vi "Idle.vi"(8 "error in":errorcluster, 11 "VISA Interface in":refnum<class "VISA Interface.lvclass">) -> (0 "error out":errorcluster, 3 "VISA Interface out":refnum<class "VISA Interface.lvclass">)   [LabVIEW 2020, in "Plugin Instrument Driver.lvlib" / "VISA Interface.lvclass"]
doc: "Clears the buffer until all other configured Plugins are completed executing their initialize states"
uses:
  VISA Interface.lvclass
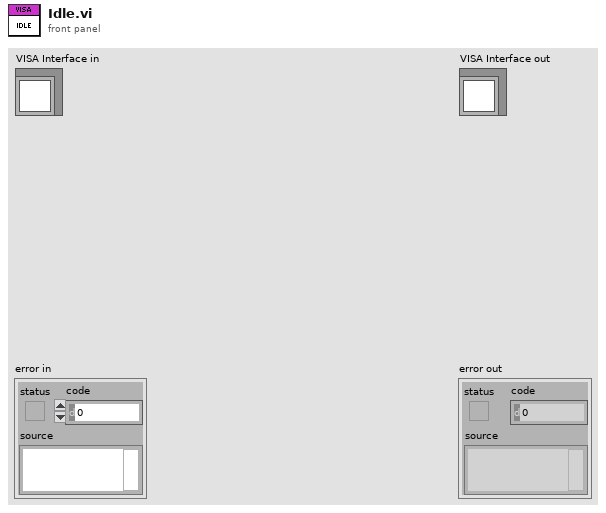
[diagram p1: front panel]
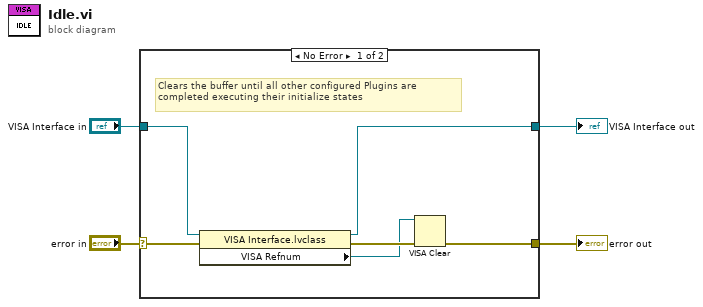
[diagram p0: block diagram]
diagram:
  n1 = case shown="No Error" "error in" {
    selector: "error in" -> [w8 w12]
    tunnel: [w7 w12] -> w3
    tunnel: [w5 w11] -> w1
    tunnel: "VISA Interface in" -> [w6 w11]
    frame No Error {
      # "Clears the buffer until all other configured Plugins are completed executing their initialize states"
      n2 = property class="VISA Interface.lvclass"(reference=w6, error in=w8) -> (reference out=w5:refnum<class "VISA Interface.lvclass">, error out=w10:errorcluster, "VISA Refnum"=w9:refnum<visa-resource-name>)
      n3 = VISA Clear(VISA resource name=w9, error in (no error)=w10) -> (error out=w7:errorcluster)  [unwired: 1 out]
    }
    frame Error {
    }
  }
  "error out" <- w3
  "VISA Interface out" <- w1
